vi "U6 Efunction Loop Example.vi"() -> (0 "error out":errorcluster)   [LabVIEW 2021]
panel:
  in  "FirstFound":bool=TRUE
  in  "Address":string="1"
  out "AIN1 Voltage":dbl format="%.6f"
  in  "stop":bool
  in  "Interval (ms)":u32=500
  out "FIO1 State In":bool
  in  "DAC0 Voltage":dbl format="%.3f"
  in  "FIO2 State Out":bool
  out "Error Message":string
  out "AIN0 Voltage":dbl format="%.6f"
  # "Sets DAC0, sets FIO2, reads AIN0, reads AIN1, and reads FIO1."
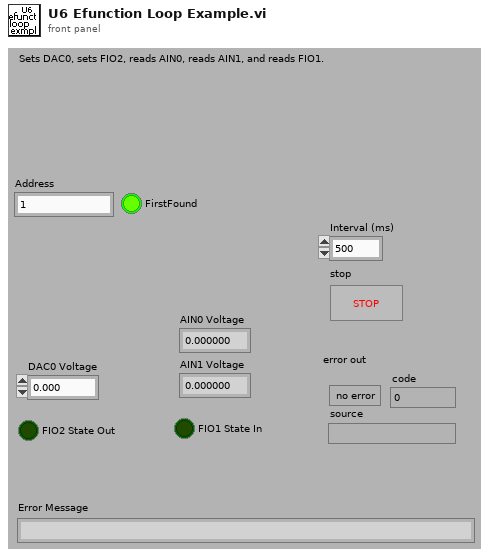
[diagram p1: front panel]
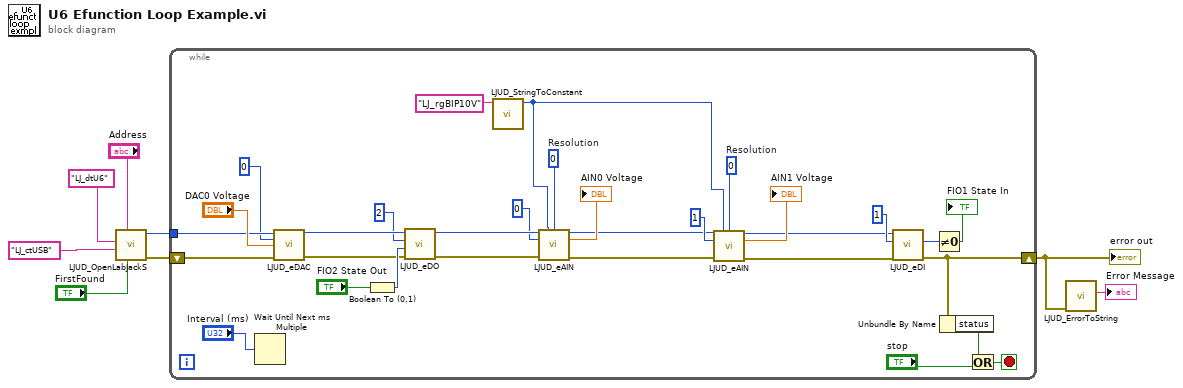
[diagram p0: block diagram]
diagram:
  n1 = call "LJUD_OpenLabJackS.vi"("FirstFound"="FirstFound", "Address"="Address", "ConnectionType"="LJ_ctUSB", "DeviceType"="LJ_dtU6") -> ("error out"=w4:errorcluster, "Handle"=w6:i32)  [unwired: 5 in, 1 out]
  n2 = while {
    shift-left: w4 -> [w20]
    shift-right: [w21] -> w5
    tunnel: w6 -> [w34]
    stop <- w23 stop-if-true
    w13 = 0  # Resolution
    w14 = 0  # Resolution
    n3 = Wait Until Next ms Multiple(millisecond multiple="Interval (ms)") -> ()  [unwired: 1 out]
    n4 = call "LJUD_eDAC.vi"("Handle In"=w34, "Channel"=0, "Voltage"="DAC0 Voltage", "error in"=w20) -> ("Handle Out"=w32:i32, "error out"=w33:errorcluster)  [unwired: 10 in]
    n5 = Boolean To (0,1)(Boolean="FIO2 State Out") -> (0, 1=w37:i16)
    n6 = call "LJUD_eDO.vi"("error in"=w33, "State"=w37, "Channel"=2, "Handle In"=w32) -> ("error out"=w31:errorcluster, "Handle Out"=w30:i32)  [unwired: 6 in]
    n7 = call "LJUD_StringToConstant.vi"("String"="LJ_rgBIP10V") -> ("Constant Number"=w9:i32)  [unwired: 9 in, 1 out]
    n8 = call "LJUD_eAIN.vi"("Handle In"=w30, "Range"=w9, "Resolution"=w14, "ChannelP"=0, "error in"=w31) -> ("Handle Out"=w12:i32, "Voltage"=→"AIN0 Voltage":dbl, "error out"=w17:errorcluster)  [unwired: 8 in]
    n9 = call "LJUD_eAIN.vi"("Handle In"=w12, "Range"=w9, "Resolution"=w13, "ChannelP"=1, "error in"=w17) -> ("Handle Out"=w11:i32, "Voltage"=→"AIN1 Voltage":dbl, "error out"=w16:errorcluster)  [unwired: 8 in]
    n10 = call "LJUD_eDI.vi"("error in"=w16, "Channel"=1, "Handle In"=w11) -> ("error out"=w21:errorcluster, "State"=w38:i32)  [unwired: 6 in, 1 out]
    n11 = Not Equal To 0?(x=w38) -> (x != 0?=→"FIO1 State In":bool)
    n12 = Unbundle By Name(w21) -> ("status"=w22:bool)
    n13 = Or(x=w22, y="stop") -> (x .or. y?=w23:bool)
  }
  "error out" <- w5
  n14 = call "LJUD_ErrorToString.vi"("error in"=w5) -> ("String"=→"Error Message":string)  [unwired: 10 in]
